vi "Configure Trigger (CAN).vi"(0 "VISA resource name":refnum<visa-resource-name>, 1 "Identifier":T2={"ID Mode (0: Standard)"=0, "ID Value (XXXXXXXXXXX)"="XXXXXXXXXXX"} {"ID Mode (0: Standard)" items=["Standard", "Extended"]}, 2 "Data":T1={"Data Size (1)"=1, "Data Value (XXXXXXXX)"="XXXXXXXX"}, 5 "Trigger Source (9: Bus 1)":u16(ring)=9 items=["Bus 1"=9, "Bus 2"=10, "Bus 3"=11, "Bus 4"=12], 7 "Condition (0: Start of Frame)":u16(ring) items=["Start of Frame", "Type of Frame", "Identifier", "Data", "ID & Data", "End of Frame", "Missing Ack"], 9 "Frame Type (0: Data)":u16(ring) items=["Data", "Remote", "Error", "Overload"], 11 "error in (no error)":errorcluster, 12 "Direction (2: Do Not Care)":u16(ring)=2 items=["Read", "Write", "Do Not Care"], 13 "Qualifier (0: Less Than)":u16(ring) items=["Less Than", "More Than", "Equal", "Not Equal", "Less Than or Equal", "More Than or Equal"]) -> (4 "VISA resource name out":refnum<visa-resource-name>, 15 "error out":errorcluster)   [LabVIEW 2016, in "Tektronix DPO MSO 2000 4000 Series.lvlib"]
doc: "Configures CAN trigger settings for an oscilloscope."
uses:
  Tektronix DPO MSO 2000 4000 Series.lvlib
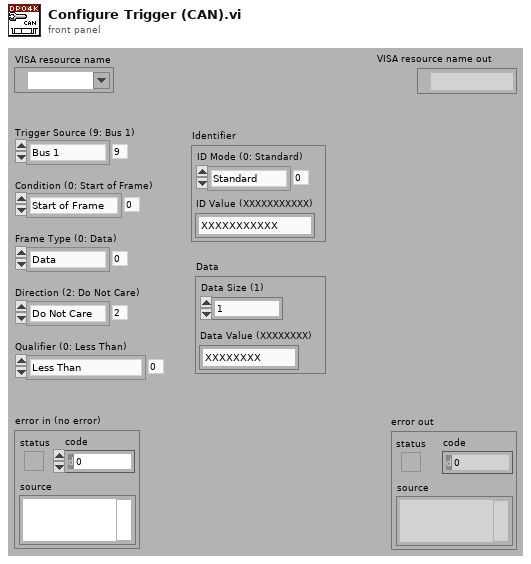
[diagram p1: front panel]
types:
  T1 = cluster{"Data Size (1)":i32, "Data Value (XXXXXXXX)":string}
  T2 = cluster{"ID Mode (0: Standard)":u16, "ID Value (XXXXXXXXXXX)":string}
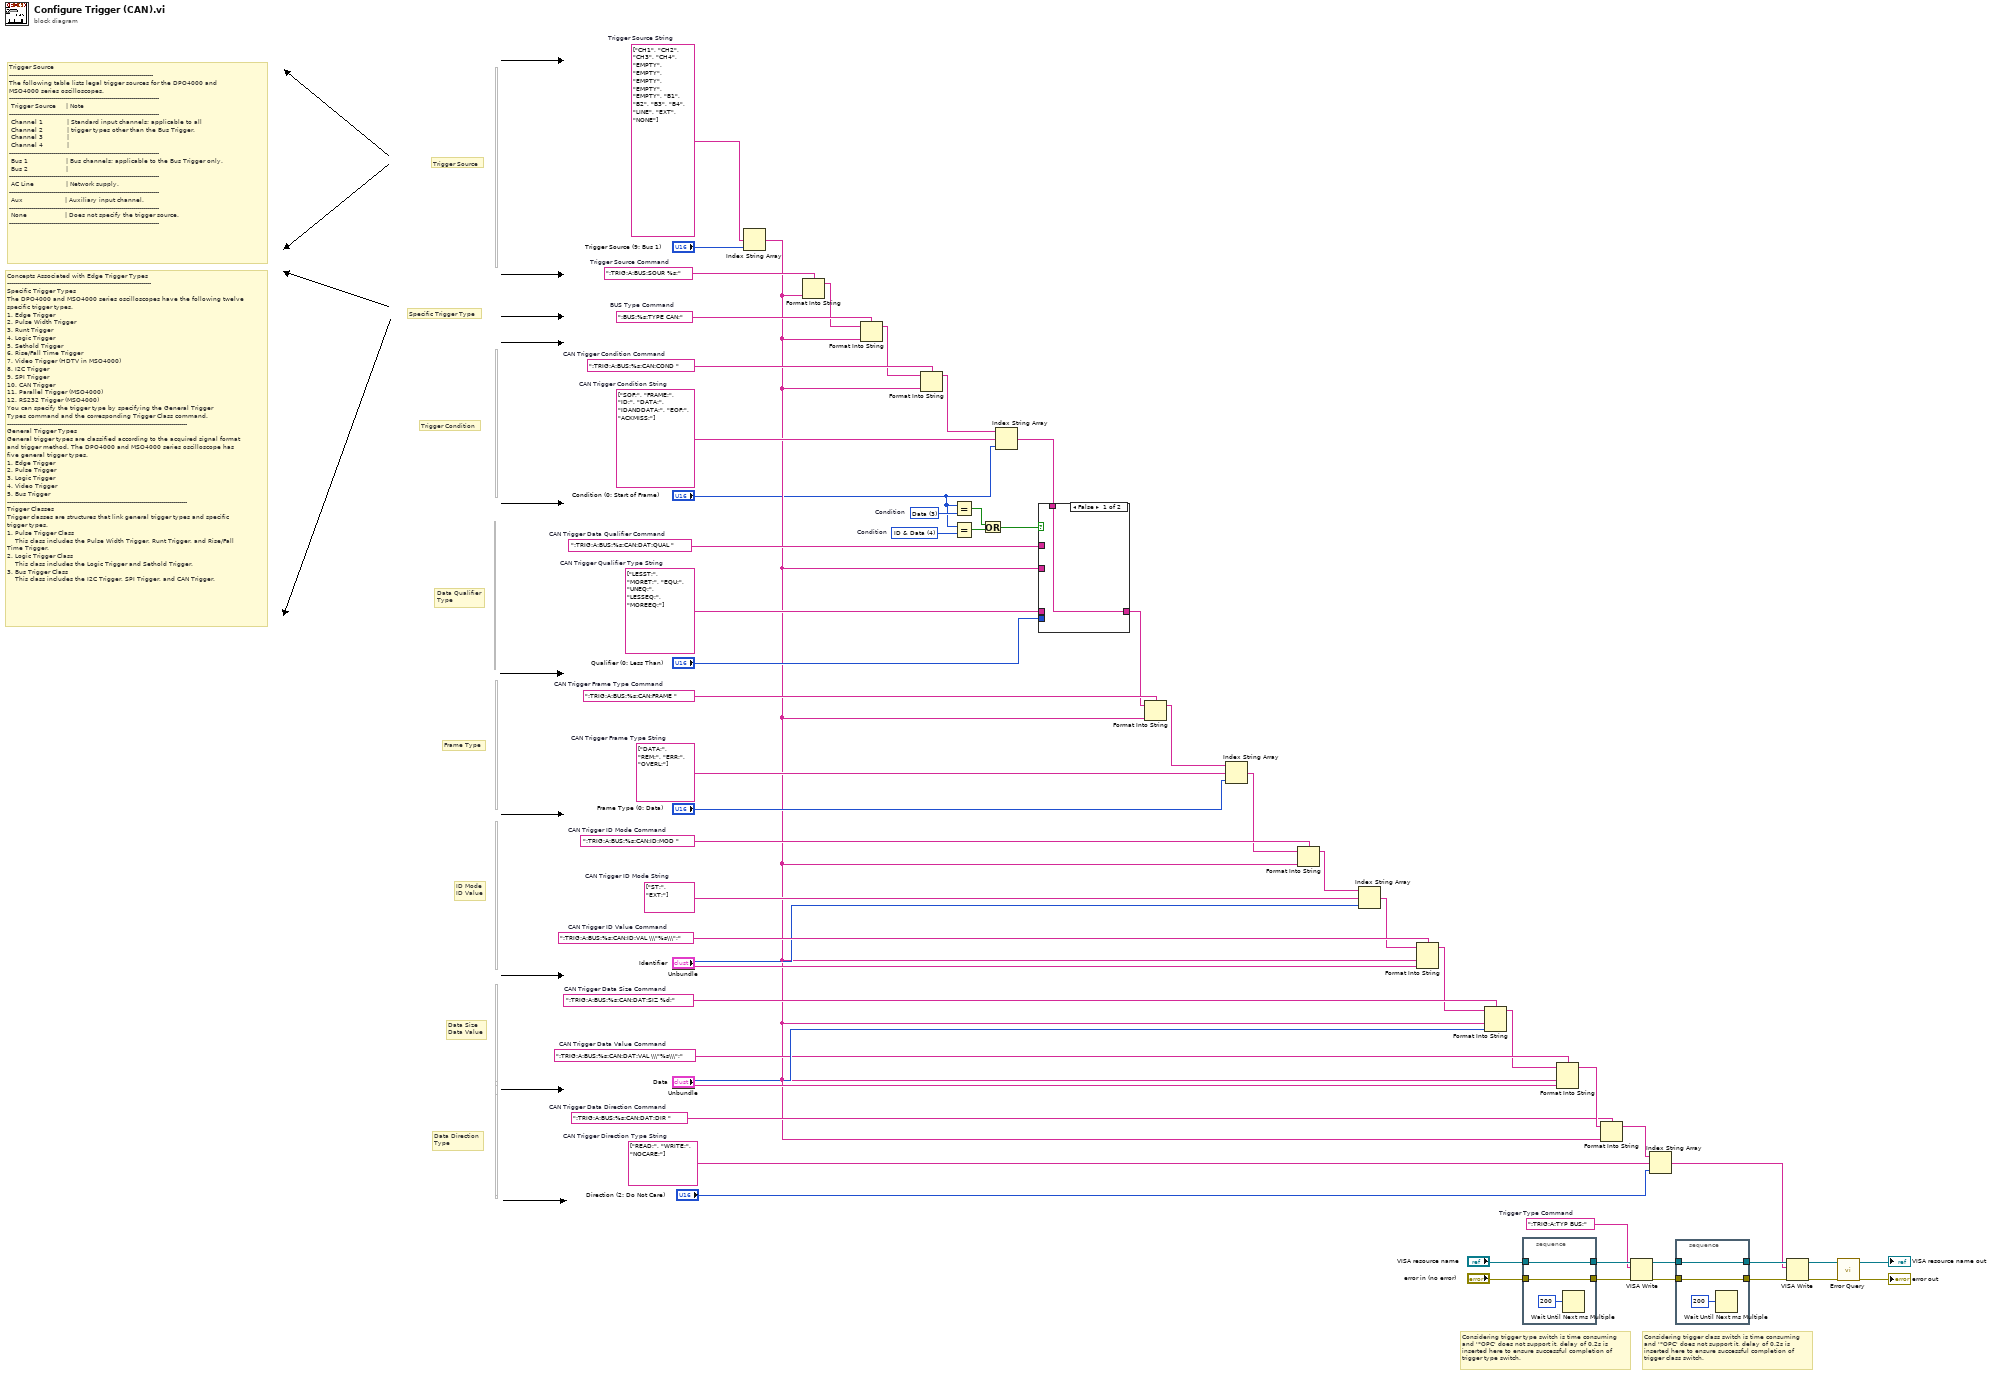
[diagram p0: block diagram]
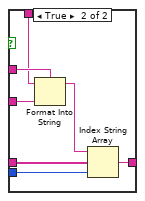
[diagram p2: hidden frame]
diagram:
  w4 = u16 4 items=["Start of Frame", "Type of Frame", "Identifier", "Data", "ID & Data", "End of Frame", "Missing Ack"]  # Condition
  w6 = u16 3 items=["Start of Frame", "Type of Frame", "Identifier", "Data", "ID & Data", "End of Frame", "Missing Ack"]  # Condition
  w12 = string[] ["LESST;", "MORET;", "EQU;", "UNEQ;", "LESSEQ;", "MOREEQ;"]  # CAN Trigger Qualifier Type String
  w15 = string[] ["READ;", "WRITE;", "NOCARE;"]  # CAN Trigger Direction Type String
  w13 = ":TRIG:A:BUS:%s:CAN:DAT:QUAL "  # CAN Trigger Data Qualifier Command
  w17 = ":TRIG:A:BUS:%s:CAN:DAT:DIR "  # CAN Trigger Data Direction Command
  w27 = string[] ["CH1", "CH2", "CH3", "CH4", "EMPTY", "EMPTY", "EMPTY", "EMPTY", "EMPTY", "B1", "B2", "B3", "B4", "LINE", "EXT", "NONE"]  # Trigger Source String
  w26 = ":TRIG:A:BUS:SOUR %s;"  # Trigger Source Command
  w35 = ":TRIG:A:TYP BUS;"  # Trigger Type Command
  w39 = ":TRIG:A:BUS:%s:CAN:DAT:VAL \\\"%s\\\";"  # CAN Trigger Data Value Command
  w44 = ":TRIG:A:BUS:%s:CAN:DAT:SIZ %d;"  # CAN Trigger Data Size Command
  w47 = ":TRIG:A:BUS:%s:CAN:ID:VAL \\\"%s\\\";"  # CAN Trigger ID Value Command
  w49 = string[] ["ST;", "EXT;"]  # CAN Trigger ID Mode String
  w51 = ":TRIG:A:BUS:%s:CAN:ID:MOD "  # CAN Trigger ID Mode Command
  w54 = string[] ["DATA;", "REM;", "ERR;", "OVERL;"]  # CAN Trigger Frame Type String
  w56 = ":TRIG:A:BUS:%s:CAN:FRAME "  # CAN Trigger Frame Type Command
  w57 = string[] ["SOF;", "FRAME;", "ID;", "DATA;", "IDANDDATA;", "EOF;", "ACKMISS;"]  # CAN Trigger Condition String
  w59 = ":TRIG:A:BUS:%s:CAN:COND "  # CAN Trigger Condition Command
  w25 = ":BUS:%s:TYPE CAN;"  # BUS Type Command
  # "Data Qualifier\nType"
  # "Data Direction\nType"
  # "Concepts Associated with Edge Trigger Types\n------------------------------------------------------------------------\nSpecific Trigger Types\nThe DPO4000 and MSO4000 series oscilloscopes have the following twelve specific trigger types.\n1. Edge Trigger\n2. Pulse Width Trigger\n3. Runt Trigger\n4. Logic Trigger\n5. Sethold Trigger\n6. Rise/Fall Time Trigger\n7. Video Trigger (HDTV in MSO4000)\n8. I2C Trigger\n9. SPI Trigger\n10. CAN Trigger\n11. Parallel Trigger (MSO4000)\n12. RS232 Trigger (MSO4000)\nYou can specify the trigger type by specifying the General Trigger \nTypes command and the corresponding Trigger Class command.\n------------------------------------------------------------------------------------------\nGeneral Trigger Types \nGeneral trigger types are classified according to the acquired signal format and trigger method. The DPO4000 and MSO4000 series oscilloscope has five general trigger types.\n1. Edge Trigger\n2. Pulse Trigger\n3. Logic Trigger\n4. Video Trigger\n5. Bus Trigger\n------------------------------------------------------------------------------------------\nTrigger Classes\nTrigger classes are structures that link general trigger types and specific trigger types.\n1. Pulse Trigger Class\n    This class includes the Pulse Width Trigger, Runt Trigger, and Rise/Fall Time Trigger.\n2. Logic Trigger Class\n    This class includes the Logic Trigger and Sethold Trigger.\n3. Bus Trigger Class\n    This class includes the I2C Trigger, SPI Trigger, and CAN Trigger."
  # "Trigger Source\n------------------------------------------------------------------------\nThe following table lists legal trigger sources for the DPO4000 and MSO4000 series oscilloscopes.\n---------------------------------------------------------------------------\n Trigger Source     | Note                                                           \n---------------------------------------------------------------------------\n Channel 1            | Standard input channels; applicable to all      \n Channel 2            | trigger types other than the Bus Trigger.         \n Channel 3            |     \n Channel 4            |\n---------------------------------------------------------------------------\n Bus 1                   | Bus channels; applicable to the Bus Trigger only.\n Bus 2                   | \n---------------------------------------------------------------------------\n AC Line                | Network supply.\n---------------------------------------------------------------------------\n Aux                     | Auxiliary input channel.\n---------------------------------------------------------------------------\n None                   | Does not specify the trigger source.\n---------------------------------------------------------------------------"
  # "Data Size\nData Value"
  # "ID Mode\nID Value"
  # "Frame Type"
  # "Trigger Condition"
  # "Specific Trigger Type"
  # "Trigger Source"
  # "Considering trigger class switch is time consuming\nand '*OPC' does not support it, delay of 0.2s is \ninserted here to ensure successful completion of\ntrigger class switch."
  # "Considering trigger type switch is time consuming\nand '*OPC' does not support it, delay of 0.2s is \ninserted here to ensure successful completion of\ntrigger type switch."
  n1 = Unbundle("Identifier") -> ("ID Mode (0: Standard)"=w45:u16, "ID Value (XXXXXXXXXXX)"=w46:string)
  n2 = Unbundle("Data") -> ("Data Size (1)"=w40:i32, "Data Value (XXXXXXXX)"=w41:string)
  n3 = Index String Array(1:"Trigger Source (9: Bus 1)", 2:w27) -> (0:w9:string)  [unwired: 1 in]
  n4 = Format Into String(format string=w26, w9) -> (resulting string=w23:string)  [unwired: 2 in, 1 out]
  n5 = Format Into String(format string=w25, initial string=w23, w9) -> (resulting string=w24:string)  [unwired: 1 in, 1 out]
  n6 = Format Into String(format string=w59, initial string=w24, w9) -> (resulting string=w58:string)  [unwired: 1 in, 1 out]
  n7 = Equal?(x="Condition (0: Start of Frame)", y=w6) -> (x = y?=w2:bool)
  n8 = Equal?(x="Condition (0: Start of Frame)", y=w4) -> (x = y?=w3:bool)
  n9 = Or(x=w2, y=w3) -> (x .or. y?=w1:bool)
  n10 = Index String Array(1:"Condition (0: Start of Frame)", 2:w57, 3:w58) -> (0:w10:string)
  n11 = case shown="False" w1 {
    tunnel: w13 -> [_ w67]
    tunnel: w12 -> [_ w66]
    tunnel: "Qualifier (0: Less Than)" -> [_ w65]
    tunnel: w10 -> [w61 w64]
    tunnel: w9 -> [_ w63]
    tunnel: [w61 w62] -> w8
    frame False {
    }
    frame True {
      n12 = Format Into String(format string=w67, initial string=w64, w63) -> (resulting string=w68:string)  [unwired: 1 in, 1 out]
      n13 = Index String Array(1:w65, 2:w66, 3:w68) -> (0:w62:string)
    }
  }
  n14 = Format Into String(format string=w56, initial string=w8, w9) -> (resulting string=w55:string)  [unwired: 1 in, 1 out]
  n15 = Index String Array(1:"Frame Type (0: Data)", 2:w54, 3:w55) -> (0:w50:string)
  n16 = Format Into String(format string=w51, initial string=w50, w9) -> (resulting string=w48:string)  [unwired: 1 in, 1 out]
  n17 = Index String Array(1:w45, 2:w49, 3:w48) -> (0:w28:string)
  n18 = Format Into String(format string=w47, initial string=w28, w9, w46) -> (resulting string=w43:string)  [unwired: 1 in, 1 out]
  n19 = Format Into String(format string=w44, initial string=w43, w9, w40) -> (resulting string=w38:string)  [unwired: 1 in, 1 out]
  n20 = stacked-sequence {
    tunnel: "VISA resource name" -> [w70]
    tunnel: [w70] -> w37
    tunnel: "error in (no error)" -> [w69]
    tunnel: [w69] -> w36
    frame #0 {
      n21 = Wait Until Next ms Multiple(millisecond multiple=u32 200) -> ()  [unwired: 1 out]
    }
  }
  n22 = Format Into String(format string=w39, initial string=w38, w9, w41) -> (resulting string=w18:string)  [unwired: 1 in, 1 out]
  n23 = Format Into String(format string=w17, initial string=w18, w9) -> (resulting string=w16:string)  [unwired: 1 in, 1 out]
  n24 = VISA Write(VISA resource name=w37, write buffer=w35, error in (no error)=w36) -> (VISA resource name out=w34:refnum<visa-resource-name>, error out=w33:errorcluster)  [unwired: 1 out]
  n25 = Index String Array(1:"Direction (2: Do Not Care)", 2:w15, 3:w16) -> (0:w7:string)
  n26 = stacked-sequence {
    tunnel: w34 -> [w73]
    tunnel: [w73] -> w29
    tunnel: w33 -> [w72]
    tunnel: [w72] -> w32
    frame #0 {
      n27 = Wait Until Next ms Multiple(millisecond multiple=u32 200) -> ()  [unwired: 1 out]
    }
  }
  n28 = VISA Write(VISA resource name=w29, write buffer=w7, error in (no error)=w32) -> (VISA resource name out=w31:refnum<visa-resource-name>, error out=w30:errorcluster)  [unwired: 1 out]
  n29 = call "Error Query.vi"("error in (no error)"=w30, "VISA resource name"=w31) -> ("error out"=→"error out":errorcluster, "VISA resource name out"=→"VISA resource name out":refnum<visa-resource-name>)  [unwired: 6 in, 2 out]
